vi "MGI Bezier Reflection Point.vi"(0 "Points Before[][]":dbl[][](array[numeric]) format="%.2f", 1 "Factor":dbl format="%.2f", 2 "psum Before[]":dbl[](array[numeric]) format="%.2f", 3 "f Values Before[]":dbl[](array[numeric]) format="%.2f", 4 "High Index":u32=1) -> (6 "Points After[][]":dbl[][](array[numeric]) format="%.2f", 7 "psum After[]":dbl[](array[numeric]) format="%.2f", 8 "New f Value":dbl format="%.2f", 9 "f Values After[]":dbl[](array[numeric]) format="%.2f")   [LabVIEW 2016]
doc: "Internal Functional Global VI used by Bezier Optimizer.\n\nAuthored by David A. Moore\nsupport@mooregoodideas.com\nwww.mooregoodideas.com\n\nCopyright (c) 2010, Moore Good Ideas, Inc.\n\nAll rights reserved.\n\nRedistribution and use in source and binary forms, with or without modification, are permitted provided that the following conditions are met:\n\n * Redistributions of source code must retain the above copyright notice, this list of conditions and the following disclaimer.\n * Redistributions in binary form must reproduce the above copyright notice, this list of conditions and the following disclaimer in the documentation and/or other materials provided with the distribution.\n * Neither the name of Moore Good Ideas, Inc. nor the names of its contributors may be used to endorse or promote products derived from this software without specific prior written permission.\n\nTHIS SOFTWARE IS PROVIDED BY THE COPYRIGHT HOLDERS AND CONTRIBUTORS \"AS IS\" AND ANY EXPRESS OR IMPLIED WARRANTIES, INCLUDING, BUT NOT LIMITED TO, THE IMPLIED WARRANTIES OF MERCHANTABILITY AND FITNESS FOR A PARTICULAR PURPOSE ARE DISCLAIMED. IN NO EVENT SHALL THE COPYRIGHT OWNER OR CONTRIBUTORS BE LIABLE FOR ANY DIRECT, INDIRECT, INCIDENTAL, SPECIAL, EXEMPLARY, OR CONSEQUENTIAL DAMAGES (INCLUDING, BUT NOT LIMITED TO, PROCUREMENT OF SUBSTITUTE GOODS OR SERVICES; LOSS OF USE, DATA, OR PROFITS; OR BUSINESS INTERRUPTION) HOWEVER CAUSED AND ON ANY THEORY OF LIABILITY, WHETHER IN CONTRACT, STRICT LIABILITY, OR TORT (INCLUDING NEGLIGENCE OR OTHERWISE) ARISING IN ANY WAY OUT OF THE USE OF THIS SOFTWARE, EVEN IF ADVISED OF THE POSSIBILITY OF SUCH DAMAGE.i"
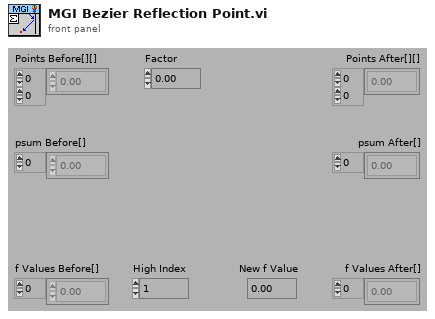
[diagram p1: front panel]
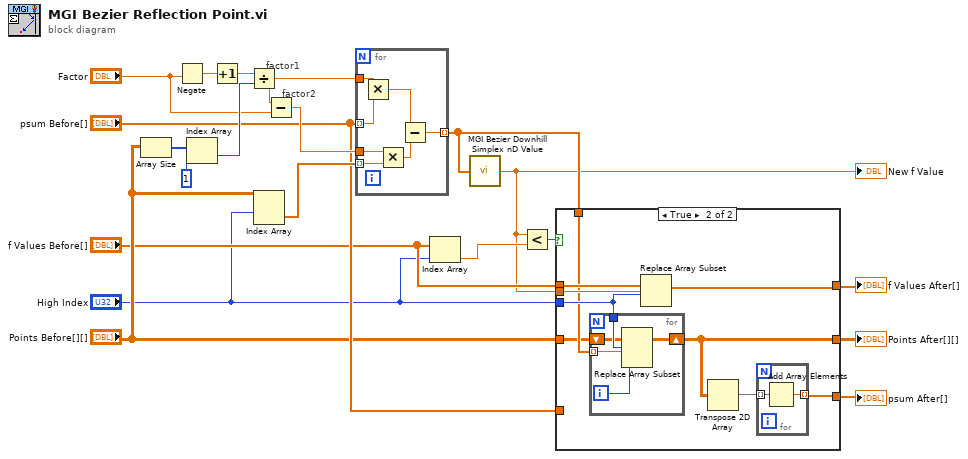
[diagram p0: block diagram]
diagram:
  # "factor2"
  # "factor1"
  n1 = Array Size(array="Points Before[][]") -> (size(s)=w20:i32[])
  n2 = Negate(x="Factor") -> (-x=w18:dbl)
  n3 = Index Array(array=w20, index=1) -> (element=w16:i32)
  n4 = Increment(x=w18) -> (x+1=w17:dbl)
  n5 = Divide(x=w17, y=w16) -> (x/y=w15:dbl)
  n6 = Index Array(array="Points Before[][]", index (row)="High Index") -> (element=w13:dbl[])  [unwired: 1 in]
  n7 = Subtract(x=w15, y="Factor") -> (x-y=w12:dbl)
  n8 = for {
    tunnel: w15 -> [w27]
    tunnel: "psum Before[]" -> [w26] mode=indexing
    tunnel: w13 -> [w25] mode=indexing
    tunnel: w12 -> [w24]
    tunnel: [w21] -> w3 mode=indexing
    n9 = Multiply(x=w27, y=w26) -> (x*y=w23:dbl)
    n10 = Multiply(x=w24, y=w25) -> (x*y=w22:dbl)
    n11 = Subtract(x=w23, y=w22) -> (x-y=w21:dbl)
  }
  n12 = Index Array(array="f Values Before[]", index="High Index") -> (element=w7:dbl)
  n13 = call <userlib>:"MGI Bezier Downhill Simplex nD Value.vi"("x[]"=w3) -> ("f(x)"=w1:dbl)
  "New f Value" <- w1
  n14 = Less?(x=w1, y=w7) -> (x < y?=w2:bool)
  n15 = case shown="True" w2 {
    tunnel: "psum Before[]" -> [w30 _]
    tunnel: [w30 w33] -> w10
    tunnel: "Points Before[][]" -> [w29 w32]
    tunnel: [w29 w31] -> w8
    tunnel: "f Values Before[]" -> [w28 w39]
    tunnel: [w28 w37] -> w5
    tunnel: "High Index" -> [_ w36]
    tunnel: w1 -> [_ w38]
    tunnel: w3 -> [_ w35]
    frame False {
    }
    frame True {
      n16 = for {
        tunnel: w36 -> [w45]
        tunnel: w35 -> [w44] mode=indexing
        shift-right: [w42] -> w31
        shift-left: w32 -> [w43]
        i -> [w46]
        n17 = Replace Array Subset(array=w43, new element=w44, index (row)=w45, index (col)=w46) -> (w42:dbl[][])
      }
      n18 = Replace Array Subset(array=w39, new element=w38, index=w36) -> (w37:dbl[])
      n19 = Transpose 2D Array(2D array=w31) -> (transposed array=w34:dbl[][])
      n20 = for {
        tunnel: w34 -> [w41] mode=indexing
        tunnel: [w40] -> w33 mode=indexing
        n21 = Add Array Elements(numeric array=w41) -> (sum=w40:dbl)
      }
    }
  }
  "Points After[][]" <- w8
  "psum After[]" <- w10
  "f Values After[]" <- w5
